vi "ES_Packet_Encode_and_Decode_Test.vi"() -> ()   [LabVIEW 2017]
uses:
  Classes/ADCP.lvclass
panel:
  out "ES Packet out":T1
  in  "ES Packet In":T1
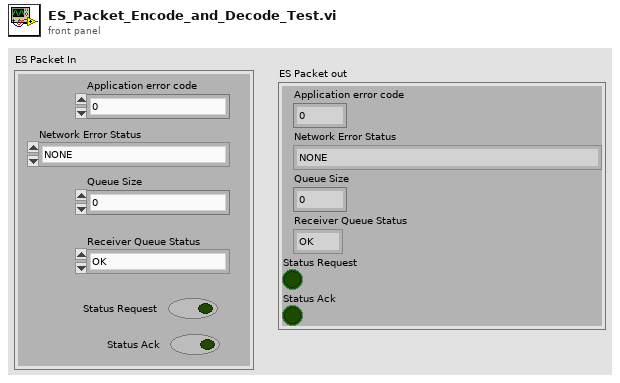
[diagram p1: front panel]
types:
  T1 = cluster{"Application error code":u16, "Network Error Status":enum16{"NONE", "CONNECTION_ALREADY_OPEN", "CONNECTION_ALREADY_CLOSED", "INVALID_FRAME_REQUEST"}, "Queue Size":u16, "Receiver Queue Status":enum16{"OK", "EMPTY", "FULL"}, "Status Request":bool, "Status Ack":bool}
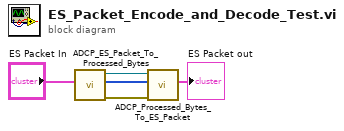
[diagram p0: block diagram]
diagram:
  n1 = call "ADCP_ES_Packet_To_Processed_Bytes.vi"("ES Packet In"="ES Packet In") -> ("error out"=w3:errorcluster, "Processed Packet Bytes"=w4:u8[], "ADCP Out"=w5:refnum<class "ADCP.lvclass">)  [unwired: 8 in]
  n2 = call "ADCP_Processed_Bytes_To_ES_Packet.vi"("error in (no error)"=w3, "Processed Packet Bytes"=w4, "ADCP In"=w5) -> ("ES Packet out"=→"ES Packet out":T1)  [unwired: 6 in, 2 out]
